vi "Create NI 9474 - Digital Output.vi"(8 "error in":errorcluster, 11 "channel settings":T1[](array[typedef])) -> (0 "error out":errorcluster, 3 "NI 9474 out":refnum<class "NI 9474.lvclass">)   [LabVIEW 2020, in "Scan Engine Scripting.lvlib" / "NI 9474.lvclass"]
doc: "Creates and configures an instance of a NI-9474 digital output module that can be used to set a slot in a Scan Engine custom device chassis."
uses:
  NI 9474.lvclass
  Mode Classes/Controls/digital channel settings.ctl
  Mode Classes/Digital Output Mode/Digital Output Mode.lvclass
  C:/jenkins/workspace/ercat-custom-device_release_20.4/Custom Device Source/Scripting/Modules/Mode Classes/Mode/Mode.lvclass
  3c9433b2-50ab-4334-8be8-e7cf6d60bbc5.vi
  Scan Engine Scripting.lvlib
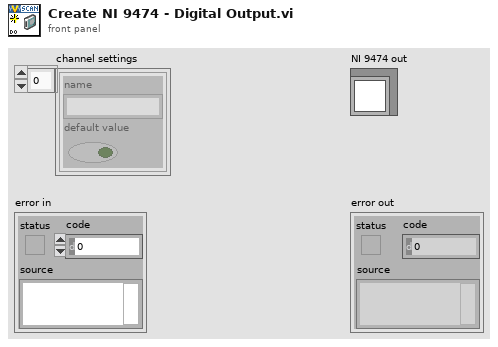
[diagram p1: front panel]
types:
  T1 = typedef "Scan Engine Scripting.lvlib/digital channel settings.ctl" = cluster{"name":string, "default value":bool}
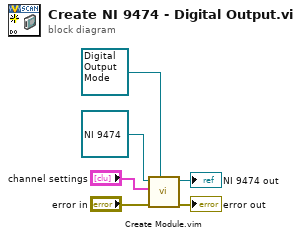
[diagram p0: block diagram]
diagram:
  n1 = call "Create Module.vim"("mode"=refnum<class "Digital Output Mode.lvclass"> refnum ("Scan Engine Scripting.lvlib:Digital Output Mode.lvclass"), "error in"="error in", "channel settings"="channel settings", "module in"=refnum<class "NI 9474.lvclass"> refnum ("NI 9474 in")) -> ("error out"=→"error out":errorcluster, "module out"=→"NI 9474 out":refnum<class "NI 9474.lvclass">)  [unwired: 6 in]
